vi "H5Sget_select_bounds.vi"(6 "error in (no error)":errorcluster, 9 "HDF5 Space Ref":T1) -> (0 "error out":errorcluster, 1 "End":i32[](array[numeric]), 2 "Start":i32[](array[numeric]), 3 "HDF5 Ref out":T1)   [LabVIEW 2017]
doc: "Gets the bounding box containing the current selection."
uses:
  <vilib>/UPVI/lvhdf5/library.llb/HDF5 Ref.ctl
  <vilib>/UPVI/lvhdf5/common.llb/U64 to I32 Array.vi
  <vilib>/UPVI/lvhdf5/hdf5.dll
panel:
  # "LVHDF5 Toolkit\nCopyright (c) 2005-2013 by Jason D. Sommerville\nCopyright (c) 2014 by UPVI, LLC.\n\nThis use and distribution of this file is governed by the terms found in \nLICENSE.txt distributed with this toolkit and installed at\n <user.lib>\\_lvhdf5\\LICENSE.txt"
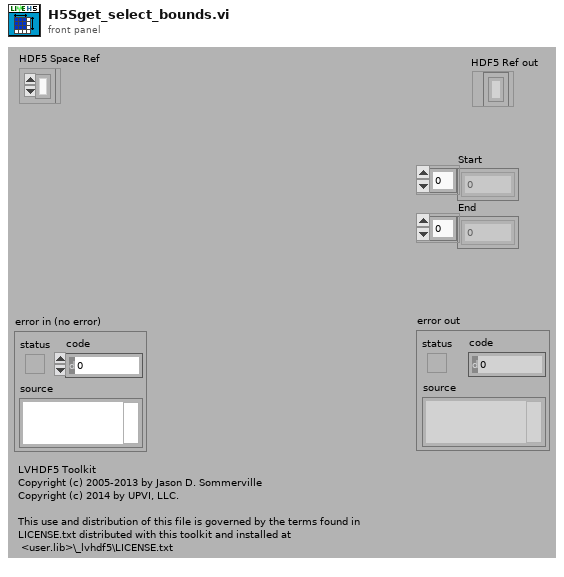
[diagram p1: front panel]
types:
  T1 = typedef "HDF5 Ref.ctl" = refnum<k1>
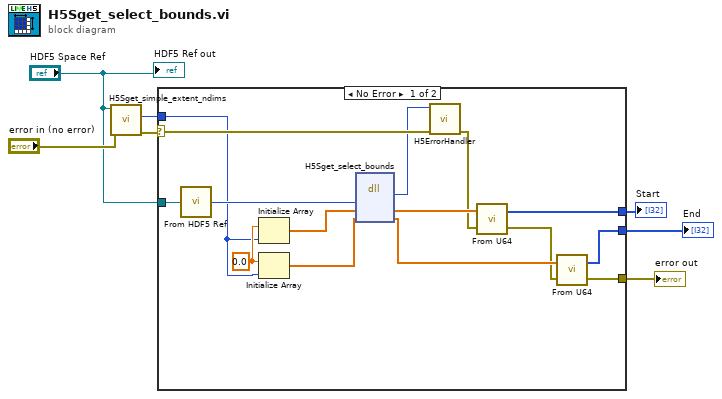
[diagram p0: block diagram]
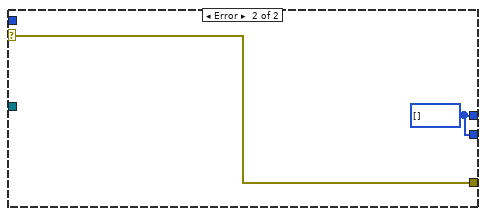
[diagram p2: hidden frame]
diagram:
  n1 = call <vilib>:"H5Sget_simple_extent_ndims.vi"("error in (no error)"="error in (no error)", "HDF5 Space Ref"="HDF5 Space Ref") -> ("error out"=w5:errorcluster, "Rank"=w3:i32)  [unwired: 5 in, 1 out]
  n2 = case shown="No Error" w5 {
    selector: w5 -> [w22 w24]
    tunnel: [w10 w24] -> w7
    tunnel: "HDF5 Space Ref" -> [w21 _]
    tunnel: w3 -> [w17 _]
    tunnel: [w9 w23] -> w2
    tunnel: [w8 w23] -> w1
    frame No Error {
      w18 = 0.0 ("element")
      n3 = call <vilib>:"From HDF5 Ref.vi"("HDF5 Ref"=w21) -> ("I32"=w20:i32)
      n4 = Initialize Array(w18, w17) -> (w15:dbl[])
      n5 = Initialize Array(w18, w17) -> (w16:dbl[])
      n6 = dll-call lib="C:/Program Files/National Instruments/LabVIEW 2017/vi.lib/UPVI/lvhdf5/hdf5.dll" fn="H5Sget_select_bounds"("space_id"=w20, "start"=w15, "end"=w16) -> (w19:i32, "start"=w14:dbl[], "end"=w13:dbl[])  [unwired: 4 in, 2 out]
      n7 = call <vilib>:"H5ErrorHandler.vi"("error in (no error)"=w22, "herr_t"=w19) -> ("error out"=w11:errorcluster)  [unwired: 3 in, 4 out]
      n8 = call-poly <vilib>:"From U64.vi"("error in (no error)"=w11, "U64"=w14) -> ("error out"=w12:errorcluster, "I32"=w8:i32[])
      n9 = call-poly <vilib>:"From U64.vi"("error in (no error)"=w12, "U64"=w13) -> ("error out"=w10:errorcluster, "I32"=w9:i32[])
    }
    frame Error {
      w23 = i32[] [] ("I32")
    }
  }
  "error out" <- w7
  "End" <- w2
  "Start" <- w1
  "HDF5 Ref out" <- "HDF5 Space Ref"
